vi "Apply_Power_Control_Setpoints_15.vi"(0 "SI804.lvclass":refnum<class "SI804.lvclass">, 2 "3 JSA30 FG112\nXA01":bool, 3 "3 JSA30 FG117\nXA01":bool, 5 "error in":errorcluster) -> (14 "SI804.lvclass out":refnum<class "SI804.lvclass">, 16 "Apply D Fact":bool, 17 "Apply D Shift":bool, 19 "error out":errorcluster)   [LabVIEW 2022 SP3, in "SI804.lvclass"]
uses:
  SI804.lvclass
  SI804.lvclass/SI804.ctl
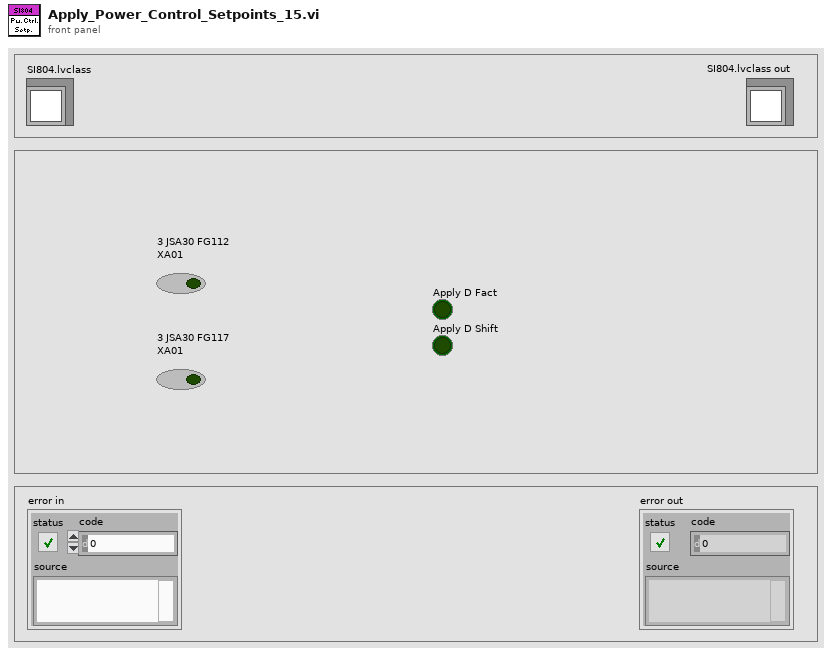
[diagram p1: front panel]
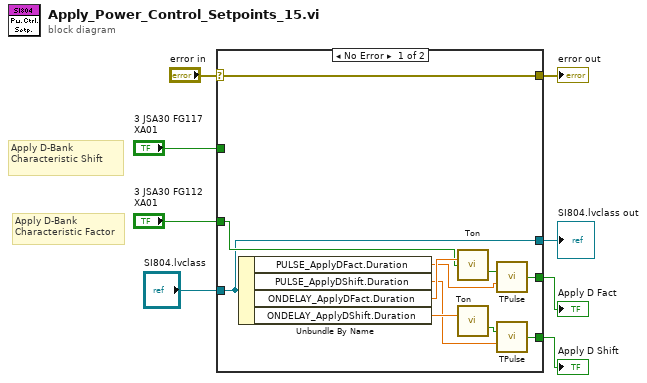
[diagram p0: block diagram]
diagram:
  # "Apply D-Bank\nCharacteristic Shift"
  # "Apply D-Bank\nCharacteristic Factor"
  n1 = case shown="No Error" "error in" {
    selector: "error in" -> [w9 w21]
    tunnel: "3 JSA30 FG112\nXA01" -> [w18 _]
    tunnel: "3 JSA30 FG117\nXA01" -> [_ _]
    tunnel: "SI804.lvclass" -> [w10 w20]
    tunnel: [w12 _] -> w4
    tunnel: [w11 _] -> w3
    tunnel: [w10 w20] -> w1
    tunnel: [w9 w21] -> w2
    frame No Error {
      n2 = Unbundle By Name(w10) -> ("PULSE_ApplyDFact.Duration"=w15:dbl, "PULSE_ApplyDShift.Duration"=w16:dbl, "ONDELAY_ApplyDFact.Duration"=w19:dbl, "ONDELAY_ApplyDShift.Duration"=w17:dbl)
      n3 = call "Ton.vi"("Ton"=w19, "input"=w18) -> ("Binary out"=w14:bool)  [unwired: 9 in, 4 out]
      n4 = call "Ton.vi"("Ton"=w17) -> ("Binary out"=w13:bool)  [unwired: 10 in, 4 out]
      n5 = call "TPulse.vi"("trigger"=w14, "TPulse"=w15) -> ("output"=w12:bool)  [unwired: 11 in, 2 out]
      n6 = call "TPulse.vi"("trigger"=w13, "TPulse"=w16) -> ("output"=w11:bool)  [unwired: 11 in, 2 out]
    }
    frame Error {
    }
  }
  "Apply D Fact" <- w4
  "Apply D Shift" <- w3
  "error out" <- w2
  "SI804.lvclass out" <- w1
